vi "Strip Quotes and Unescape.vi"(8 "error in (no error)":errorcluster, 9 "To System Encoding (T)":bool=TRUE, 11 "String":string) -> (0 "error out":errorcluster, 3 "result string":string)   [LabVIEW 2024, in "JSONtext.lvlib"]
uses:
  JSONtext.lvlib
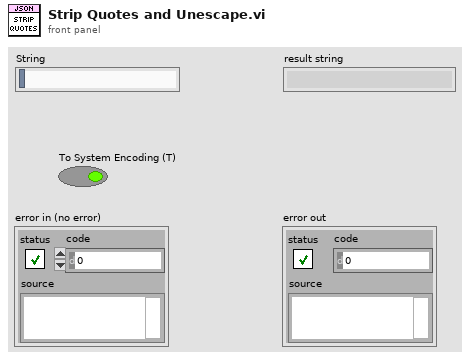
[diagram p1: front panel]
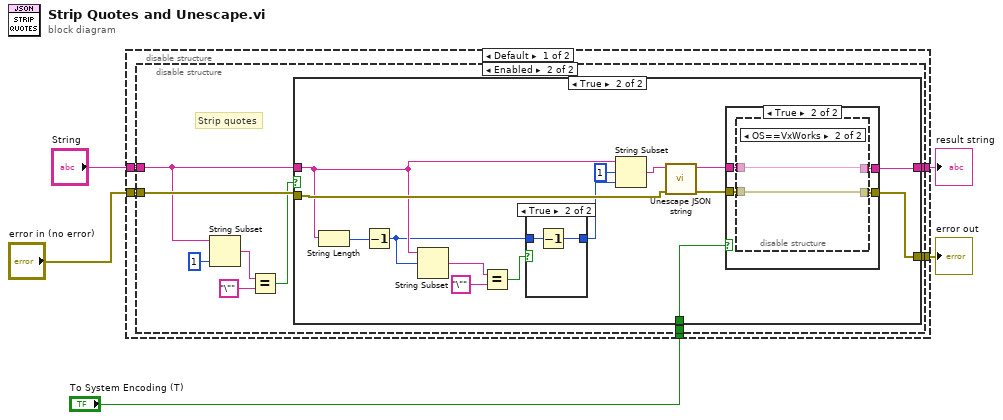
[diagram p0: block diagram]
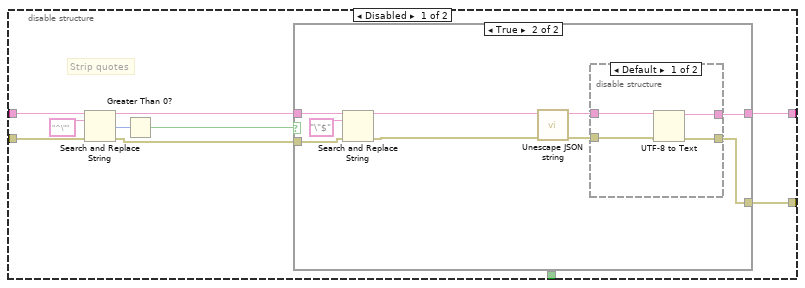
[diagram p2: hidden frame]
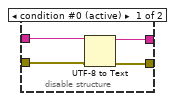
[diagram p7: hidden frame]
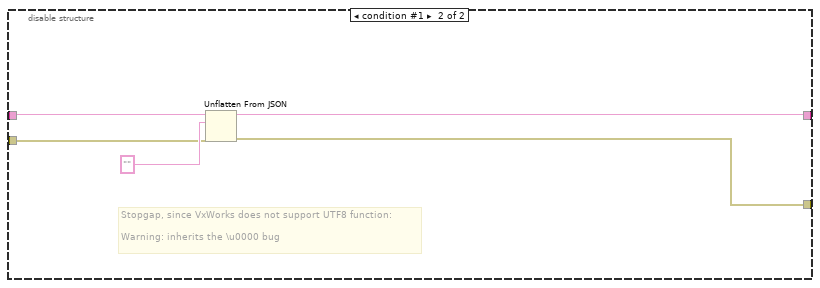
[diagram p9: hidden frame]
diagram:
  n1 = disable-structure shown="Default" {
    disable-tunnel: [w10 w78] -> w5
    disable-tunnel: "error in (no error)" -> [w9 w80]
    disable-tunnel: [w8 w79] -> w3
    disable-tunnel: "String" -> [w7 w82]
    disable-tunnel: "To System Encoding (T)" -> [w6 _]
    frame condition #0 (active) {
      n2 = disable-structure shown="Enabled" {
        disable-tunnel: [w19 w45] -> w10
        disable-tunnel: w9 -> [w17 w44]
        disable-tunnel: [w16 w43] -> w8
        disable-tunnel: w7 -> [w11 w41]
        disable-tunnel: w6 -> [_ w37]
        frame Disabled {
          # "Strip quotes"
          n3 = Search and Replace String(input string=w11, search string="^\"", error in=w17) -> (result string=w15:string, number of replacements=w13:i32, error out=w18:errorcluster)  [unwired: 5 in, 1 out]
          n4 = Greater Than 0?(x=w13) -> (x > 0?=w12:bool)
          n5 = case shown="True" w12 {
            tunnel: [w20 w22] -> w19
            tunnel: w18 -> [w20 w30]
            tunnel: [w21 w24] -> w16
            tunnel: w15 -> [w21 w29]
            frame False {
              # "Not a leading quote?   This shouldn't happen."
            }
            frame True {
              n6 = Search and Replace String(input string=w29, search string="\"$", error in=w30) -> (result string=w27:string, error out=w26:errorcluster)  [unwired: 5 in, 2 out]
              n7 = call "Unescape JSON string.vi"("error in (no error)"=w26, "Text (with JSON escapes)"=w27) -> ("error out"=w23:errorcluster, "Text (unescaped)"=w25:string)  [unwired: 8 in]
              n8 = disable-structure shown="Default" {
                disable-tunnel: w25 -> [w34 w36]
                disable-tunnel: [w33 w36] -> w24
                disable-tunnel: w23 -> [w32 w35]
                disable-tunnel: [w31 w35] -> w22
                frame condition #0 (active) {
                  n9 = UTF-8 to Text(8:w32, 11:w34) -> (0:w31:errorcluster, 3:w33:string)  [unwired: 1 in]
                }
                frame condition #1 {
                }
              }
            }
          }
        }
        frame Enabled {
          # "Strip quotes"
          n10 = String Subset(string=w41, length (rest)=1 ("length (rest)")) -> (substring=w40:string)  [unwired: 1 in]
          n11 = Equal?(x=w40, y="\"") -> (x = y?=w38:bool)
          n12 = case shown="True" w38 {
            tunnel: [w46 w58] -> w45
            tunnel: w44 -> [w46 w62]
            tunnel: [w47 w60] -> w43
            tunnel: w41 -> [w47 w54]
            tunnel: w37 -> [_ w48]
            frame False {
            }
            frame True {
              n13 = String Length(string=w54) -> (length=w55:i32)
              n14 = Decrement(x=w55) -> (x-1=w51:i32)
              n15 = String Subset(string=w54, offset (0)=w51) -> (substring=w56:string)  [unwired: 1 in]
              n16 = Equal?(x=w56, y="\"") -> (x = y?=w49:bool)
              n17 = case shown="True" w49 {
                tunnel: w51 -> [w75 w77]
                tunnel: [w75 w76] -> w50
                frame False {
                }
                frame True {
                  n18 = Decrement(x=w77) -> (x-1=w76:i32)
                }
              }
              n19 = String Subset(string=w54, offset (0)=1, length (rest)=w50) -> (substring=w52:string)
              n20 = call "Unescape JSON string.vi"("error in (no error)"=w62, "Text (with JSON escapes)"=w52) -> ("error out"=w59:errorcluster, "Text (unescaped)"=w61:string)  [unwired: 8 in]
              n21 = case shown="True" w48 {
                tunnel: w61 -> [w64 w68]
                tunnel: [w64 w67] -> w60
                tunnel: w59 -> [w63 w66]
                tunnel: [w63 w65] -> w58
                frame False {
                }
                frame True {
                  n22 = disable-structure shown="OS==VxWorks" {
                    disable-tunnel: w68 -> [w72 w74]
                    disable-tunnel: [w71 w74] -> w67
                    disable-tunnel: w66 -> [w70 w73]
                    disable-tunnel: [w69 w73] -> w65
                    frame condition #0 (active) {
                      n23 = UTF-8 to Text(8:w70, 11:w72) -> (0:w69:errorcluster, 3:w71:string)  [unwired: 1 in]
                    }
                    frame condition #1 {
                    }
                  }
                }
              }
            }
          }
        }
      }
    }
    frame condition #1 {
      # "Stopgap, since VxWorks does not support UTF8 function:\n\nWarning: inherits the \\u0000 bug"
      n24 = Unflatten From JSON(JSON string=w82, type and defaults="", error in (no error)=w80) -> (value=w79:string, error out=w78:errorcluster)  [unwired: 4 in]
    }
  }
  "error out" <- w5
  "result string" <- w3
